vi "IMAQ FPGA Camera Link Pixel Bus to Vision Pixel Bus U8x8.vi"(5 "Reset Overflow":bool, 6 "Ready for Output":bool=TRUE, 7 "Overflow In":bool, 8 "Input Valid":bool=TRUE, 9 "Frame Valid In":bool, 10 "Line Valid In":bool, 11 "Pixel Bus x8 In":cluster{"Pixels":u8[], "DV":bool[]}={"Pixels"=[0, 0, 0, 0, 0, 0, 0, 0], "DV"=[FALSE, FALSE, FALSE, FALSE, FALSE, FALSE, FALSE, FALSE]}) -> (0 "Output Valid":bool, 2 "Acquisition Overflow":bool, 3 "Vision Pixel Bus Out":T1={"Pixel Data"=[0, 0, 0, 0, 0, 0, 0, 0], "DV"=[FALSE, FALSE, FALSE, FALSE, FALSE, FALSE, FALSE, FALSE], "EOL"=FALSE, "EOI"=FALSE, "Data Type"=enum."U8 x 8"})   [LabVIEW 2017]
doc: "The Pixel Bus to Vision Pixel Bus takes the <B>Pixel Bus x8 In</B> and the timing signals (Line Valid, Frame Valid, and Input Valid) and converts them to the data structure used by Vision FPGA functions where the Line Valid and Frame Valid are part of the <B>Vision Pixel Bus Out</B> data structure.\n\nIf Ready For Output is ever False (i.e. downstream VIs are not ready for new pixel data), and this VI is about to output a valid Vision Pixel Bus, the Acquisition Overflow will assert and stay high to indicate pixel data was lost. The CameraLink pixel bus can not be slowed down, so the downstream processing VIs and transfer VIs need to ensure they can handle the CameraLink throughput to avoid missing pixels.\n\nThis VI requires a cycle to add End of Line and another cycle to add End of Image at the end of every image. This means there needs to be at least two blanking cycles between frames."
uses:
  <vilib>/visionFPGA/Controls/IMAQ FPGA Pixel Bus u8x8.ctl
  <vilib>/visionFPGA/Basics/Camera Link Acquisition/Controls/IMAQ FPGA Camera Link Pixel Bus to Vision Bus State.ctl
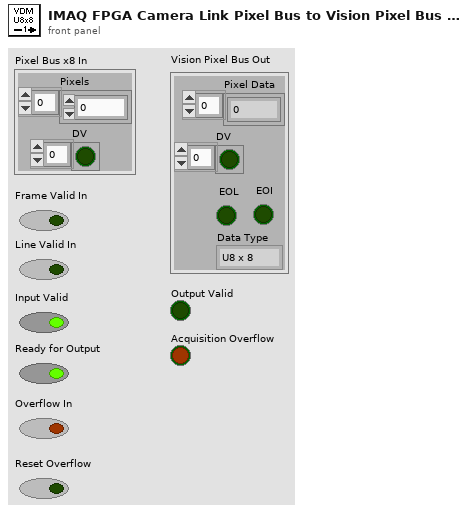
[diagram p1: front panel]
types:
  T1 = typedef "IMAQ FPGA Pixel Bus u8x8.ctl" = cluster{"Pixel Data":u8[], "DV":bool[], "EOL":bool, "EOI":bool, "Data Type":enum16{"U8 x 8"}}
  T2 = typedef "IMAQ FPGA Camera Link Pixel Bus to Vision Bus State.ctl" = enum16{"WaitForFirstPixel", "WaitForEndOfLine", "WaitForStartofNextLineOrEndOfImage", "HandleEndOfImage"}
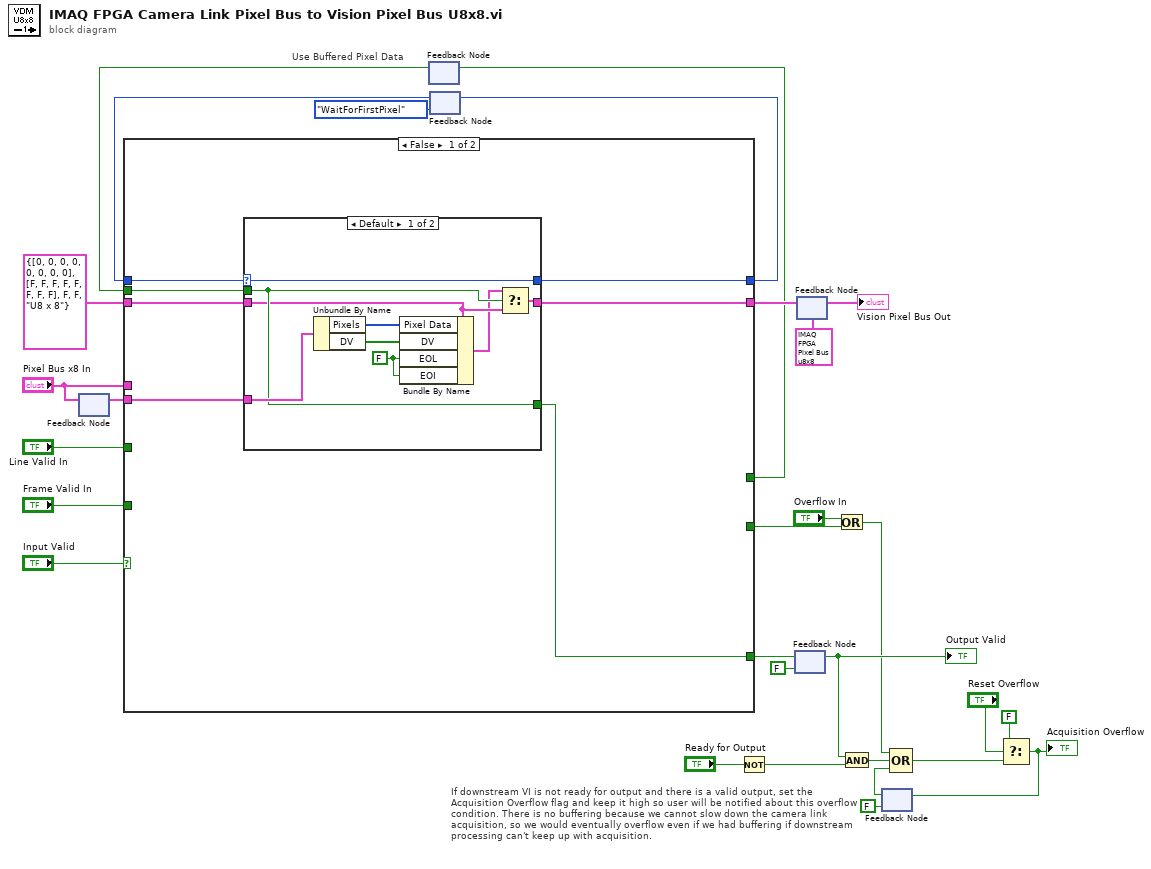
[diagram p0: block diagram]
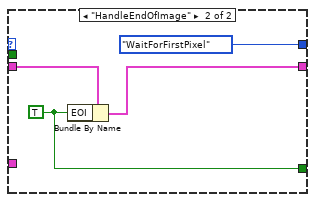
[diagram p2: hidden frame]
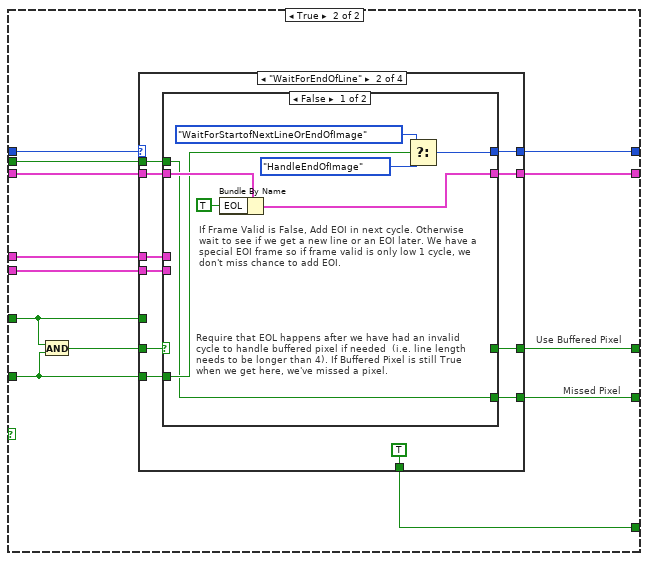
[diagram p3: hidden frame]
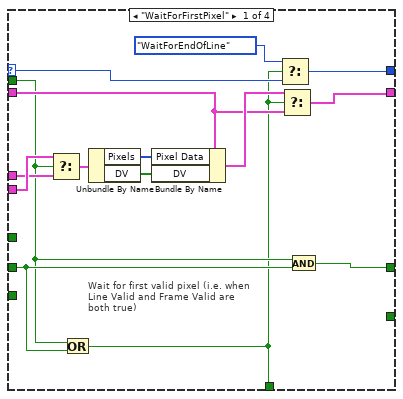
[diagram p4: hidden frame]
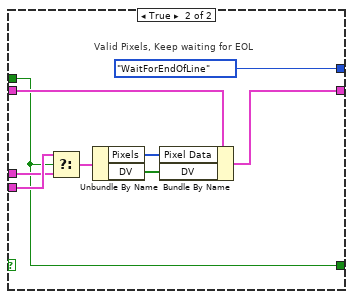
[diagram p5: hidden frame]
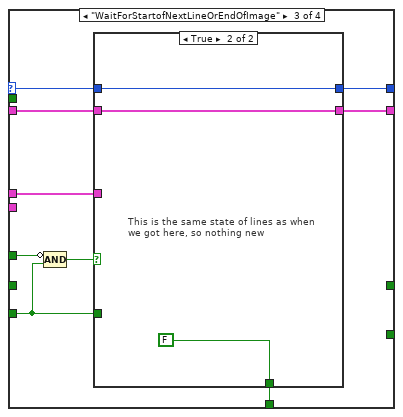
[diagram p6: hidden frame]
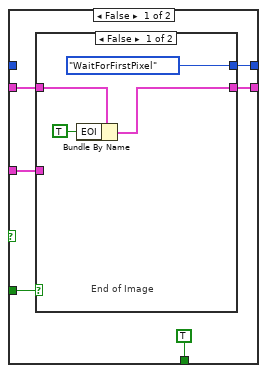
[diagram p7: hidden frame]
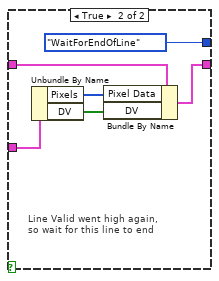
[diagram p8: hidden frame]
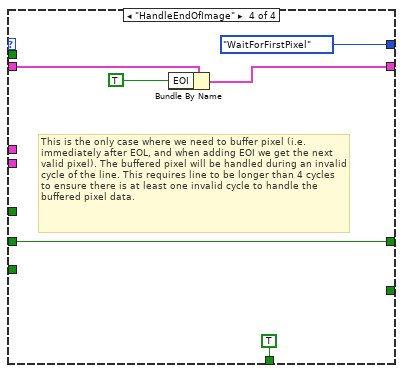
[diagram p9: hidden frame]
diagram:
  # "Use Buffered Pixel Data"
  # "If downstream VI is not ready for output and there is a valid output, set the Acquisition Overflow flag and keep it high so user will be notified about this overflow condition. There is no buffering because we cannot slow down the camera link acquisition, so we would eventually overflow even if we had buffering if downstream processing can't keep up with acquisition."
  n1 = feedback #1() -> (w5:cluster{"Pixels":u8[], "DV":bool[]})  [unwired: 1 in]
  n2 = feedback-in #1("Pixel Bus x8 In") -> ()
  n3 = feedback #2() -> (w4:bool)  [unwired: 1 in]
  n4 = feedback #3(IMAQ_FPGA_Camera_Link_Pixel_Bus_to_Vision_Bus_State."WaitForFirstPixel") -> (w9:T2)
  n5 = case shown="False" "Input Valid" {
    tunnel: [w33 w56] -> w25
    tunnel: "Line Valid In" -> [_ w58]
    tunnel: "Frame Valid In" -> [_ w57]
    tunnel: [w34 w61] -> w24
    tunnel: T1 {"Pixel Data"=[0, 0, 0, 0, 0, 0, 0, 0], "DV"=[FALSE, FALSE, FALSE, FALSE, FALSE, FALSE, FALSE, FALSE], "EOL"=FALSE, "EOI"=FALSE, "Data Type"=enum."U8 x 8"} ("Vision Pixel Bus Out") -> [w35 w62]
    tunnel: "Pixel Bus x8 In" -> [_ w60]
    tunnel: [w32 w55] -> w8
    tunnel: w9 -> [w36 w54]
    tunnel: [_ w53] -> w7
    tunnel: w5 -> [w30 w51]
    tunnel: w4 -> [w31 w52]
    tunnel: [_ w50] -> w2
    frame False {
      n6 = case shown="Default" w36 {
        selector: w36 -> [w45 _]
        tunnel: w35 -> [w39 w49]
        tunnel: [w38 w48] -> w34
        tunnel: [w40 w46] -> w33
        tunnel: [w45 IMAQ_FPGA_Camera_Link_Pixel_Bus_to_Vision_Bus_State."WaitForFirstPixel"] -> w32
        tunnel: w31 -> [w40 _]
        tunnel: w30 -> [w44 _]
        frame Default {
          w41 = FALSE ("EOL")
          n7 = Unbundle By Name(w44) -> ("Pixels"=w43:u8[], "DV"=w42:bool[])
          n8 = Bundle By Name(cluster=w39, "Pixel Data"=w43, "DV"=w42, "EOL"=w41, "EOI"=w41) -> (w37:T1)
          n9 = Select(t=w37, s=w40, f=w39) -> (s? t:f=w38:T1)
        }
        frame "HandleEndOfImage" {
          w46 = TRUE ("EOI")
          n10 = Bundle By Name(cluster=w49, "EOI"=w46) -> (w48:T1)
        }
      }
    }
    frame True {
      # "Missed Pixel"
      # "Use Buffered Pixel"
      n11 = And(x=w58, y=w57) -> (x .and. y?=w59:bool)
      n12 = case shown="\"WaitForEndOfLine\"" w54 {
        selector: w54 -> [w76 _ w112 _]
        tunnel: [w77 w84 w111 IMAQ_FPGA_Camera_Link_Pixel_Bus_to_Vision_Bus_State."WaitForFirstPixel"] -> w55
        tunnel: w57 -> [_ w83 w107 _]
        tunnel: w58 -> [_ _ w109 _]
        tunnel: w62 -> [w70 w87 w114 w138]
        tunnel: [w75 w85 w113 w137] -> w61
        tunnel: w60 -> [w68 w86 w106 _]
        tunnel: w59 -> [w65 w88 _ w134]
        tunnel: [w63 TRUE w110 TRUE] -> w56
        tunnel: [w66 w79 _ w134] -> w53
        tunnel: w52 -> [w64 w81 _ _]
        tunnel: w51 -> [w69 w80 _ _]
        tunnel: [_ w78 _ _] -> w50
        frame "WaitForFirstPixel" {
          # "Wait for first valid pixel (i.e. when Line Valid and Frame Valid are both true)"
          n13 = Select(t=w69, s=w64, f=w68) -> (s? t:f=w67:cluster{"Pixels":u8[], "DV":bool[]})
          n14 = Or(x=w64, y=w65) -> (x .or. y?=w63:bool)
          n15 = Unbundle By Name(w67) -> ("Pixels"=w74:u8[], "DV"=w73:bool[])
          n16 = Bundle By Name(cluster=w70, "Pixel Data"=w74, "DV"=w73) -> (w71:T1)
          n17 = Select(t=IMAQ_FPGA_Camera_Link_Pixel_Bus_to_Vision_Bus_State."WaitForEndOfLine", s=w63, f=w76) -> (s? t:f=w77:T2)
          n18 = Select(t=w71, s=w63, f=w70) -> (s? t:f=w75:T1)
          n19 = And(x=w64, y=w65) -> (x .and. y?=w66:bool)
        }
        frame "WaitForEndOfLine" {
          n20 = case shown="False" w88 {
            tunnel: w87 -> [w96 w105]
            tunnel: w86 -> [_ w99]
            tunnel: [w95 w102] -> w85
            tunnel: [w90 IMAQ_FPGA_Camera_Link_Pixel_Bus_to_Vision_Bus_State."WaitForEndOfLine"] -> w84
            tunnel: w83 -> [w93 _]
            tunnel: w81 -> [w89 w97]
            tunnel: w80 -> [_ w100]
            tunnel: [_ w97] -> w79
            tunnel: [w89 _] -> w78
            frame False {
              # "Require that EOL happens after we have had an invalid cycle to handle buffered pixel if needed  (i.e. line length needs to be longer than 4). If Buffered Pixel is still True when we get here, we've missed a pixel."
              # "If Frame Valid is False, Add EOI in next cycle. Otherwise wait to see if we get a new line or an EOI later. We have a special EOI frame so if frame valid is only low 1 cycle, we don't miss chance to add EOI."
              n21 = Bundle By Name(cluster=w96, "EOL"=TRUE) -> (w95:T1)
              n22 = Select(t=IMAQ_FPGA_Camera_Link_Pixel_Bus_to_Vision_Bus_State."WaitForStartofNextLineOrEndOfImage", s=w93, f=IMAQ_FPGA_Camera_Link_Pixel_Bus_to_Vision_Bus_State."HandleEndOfImage") -> (s? t:f=w90:T2)
            }
            frame True {
              # "Valid Pixels, Keep waiting for EOL"
              n23 = Select(t=w100, s=w97, f=w99) -> (s? t:f=w98:cluster{"Pixels":u8[], "DV":bool[]})
              n24 = Unbundle By Name(w98) -> ("Pixels"=w104:u8[], "DV"=w103:bool[])
              n25 = Bundle By Name(cluster=w105, "Pixel Data"=w104, "DV"=w103) -> (w102:T1)
            }
          }
        }
        frame "WaitForStartofNextLineOrEndOfImage" {
          n26 = Compound Arithmetic op=AND(invert w109, w107) -> (w108:bool)
          n27 = case shown="True" w108 {
            tunnel: w114 -> [w119 w133]
            tunnel: [w118 w133] -> w113
            tunnel: w112 -> [_ w132]
            tunnel: [w117 w132] -> w111
            tunnel: [TRUE FALSE] -> w110
            tunnel: w107 -> [w116 _]
            tunnel: w106 -> [w115 _]
            frame False {
              n28 = case shown="False" w116 {
                tunnel: w119 -> [w124 w129]
                tunnel: [w122 w125] -> w118
                tunnel: [IMAQ_FPGA_Camera_Link_Pixel_Bus_to_Vision_Bus_State."WaitForFirstPixel" IMAQ_FPGA_Camera_Link_Pixel_Bus_to_Vision_Bus_State."WaitForEndOfLine"] -> w117
                tunnel: w115 -> [_ w128]
                frame False {
                  # "End of Image"
                  n29 = Bundle By Name(cluster=w124, "EOI"=TRUE) -> (w122:T1)
                }
                frame True {
                  # "Line Valid went high again, so wait for this line to end"
                  n30 = Unbundle By Name(w128) -> ("Pixels"=w127:u8[], "DV"=w126:bool[])
                  n31 = Bundle By Name(cluster=w129, "Pixel Data"=w127, "DV"=w126) -> (w125:T1)
                }
              }
            }
            frame True {
              # "This is the same state of lines as when we got here, so nothing new"
            }
          }
        }
        frame "HandleEndOfImage" {
          # "This is the only case where we need to buffer pixel (i.e. immediately after EOL, and when adding EOI we get the next valid pixel). The buffered pixel will be handled during an invalid cycle of the line. This requires line to be longer than 4 cycles to ensure there is at least one invalid cycle to handle the buffered pixel data."
          n32 = Bundle By Name(cluster=w138, "EOI"=TRUE) -> (w137:T1)
        }
      }
    }
  }
  n33 = feedback-in #2(w7) -> ()
  n34 = feedback-in #3(w8) -> ()
  n35 = Not(x="Ready for Output") -> (.not. x?=w21:bool)
  n36 = feedback #4(FALSE) -> (w20:bool)
  "Output Valid" <- w20
  n37 = feedback-in #4(w25) -> ()
  n38 = feedback #5(T1 {"Pixel Data"=[0, 0, 0, 0, 0, 0, 0, 0], "DV"=[FALSE, FALSE, FALSE, FALSE, FALSE, FALSE, FALSE, FALSE], "EOL"=FALSE, "EOI"=FALSE, "Data Type"=enum."U8 x 8"} ("Vision Pixel Bus Out")) -> (→"Vision Pixel Bus Out":T1)
  n39 = feedback-in #5(w24) -> ()
  n40 = Or(x="Overflow In", y=w2) -> (x .or. y?=w1:bool)
  n41 = And(x=w20, y=w21) -> (x .and. y?=w19:bool)
  n42 = feedback #6(FALSE) -> (w18:bool)
  n43 = Compound Arithmetic op=OR(w1, w19, w18) -> (w13:bool)
  n44 = Select(t=FALSE, s="Reset Overflow", f=w13) -> (s? t:f=w12:bool)
  "Acquisition Overflow" <- w12
  n45 = feedback-in #6(w12) -> ()
